vi "读取打包属性.vi"(0 "引用句柄输入":refnum<k34>, 5 "组名称":string, 11 "错误输入（无错误）":errorcluster) -> (4 "测试数据":T1, 6 "数据属性":variant, 15 "错误输出":errorcluster)   [LabVIEW 2020]
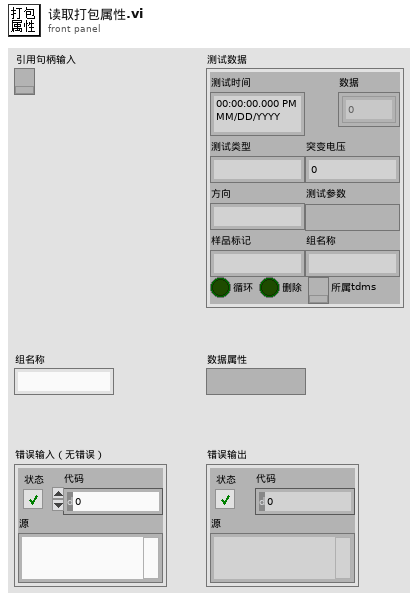
[diagram p1: front panel]
types:
  T1 = typedef "测试数据类型.ctl" = cluster{"测试时间":timestamp, "数据":dbl[][], "测试类型":string, "方向":string, "样品标记":string, "突变电压":i32, "测试参数":variant, "循环":bool, "删除":bool, "组名称":string, "所属tdms":refnum<k34>}
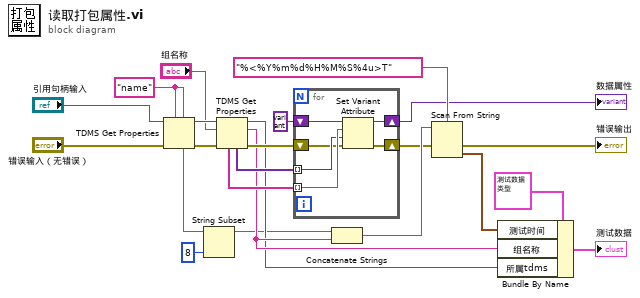
[diagram p0: block diagram]
diagram:
  w15 = "name" ("属性名称")
  n1 = TDMS Get Properties(5:w15, 7:w15, 8:"错误输入（无错误）", 11:"引用句柄输入") -> (0:w21:errorcluster, 3:w19:refnum<k34>, 4:w5:string)  [unwired: 2 in, 3 out]
  n2 = String Subset(string=w5, length (rest)=8 ("长度（剩余）")) -> (substring=w2:string)  [unwired: 1 in]
  n3 = TDMS Get Properties(8:w21, 10:"组名称", 11:w19) -> (0:w9:errorcluster, 2:w4:string, 3:w3:refnum<k34>, 4:w10:variant[], 6:w11:string[])  [unwired: 3 in, 1 out]
  n4 = for {
    tunnel: w11 -> [w29] mode=indexing
    tunnel: w10 -> [w28] mode=indexing
    shift-right: [w27] -> w12
    shift-left: variant -> [w26]
    shift-right: [w24] -> w8
    shift-left: w9 -> [w25]
    n5 = Set Variant Attribute(Variant=w26, name=w29, value=w28, error in=w25) -> (Variant out=w27:variant, error out=w24:errorcluster)  [unwired: 1 out]
  }
  "数据属性" <- w12
  n6 = Concatenate Strings(w2, w4) -> (w16:string)
  n7 = Scan From String(format string="%<%Y%m%d%H%M%S%4u>T" ("格式字符串"), input string=w16, error in=w8) -> (error out=→"错误输出":errorcluster, output 1=w6:timestamp)  [unwired: 2 in, 2 out]
  n8 = Bundle By Name(cluster=T1 {"测试时间"=timestamp(0 s since 1904-01-01), "数据"=[], "测试类型"="", "方向"="", "样品标记"="", "突变电压"=0, "测试参数"=variant(string ""), "循环"=FALSE, "删除"=FALSE, "组名称"="", "所属tdms"=refnum} ("测试数据"), "测试时间"=w6, "组名称"=w4, "所属tdms"=w3) -> (→"测试数据":T1)
